vi "GUID.vi"() -> (3 "trimmed string":string caption="GUID")   [LabVIEW 2018]
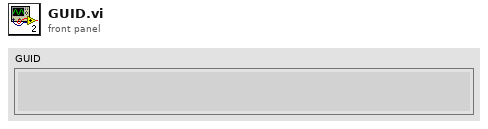
[diagram p1: front panel]
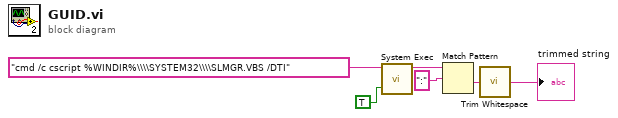
[diagram p0: block diagram]
diagram:
  n1 = call <vilib>:"System Exec.vi"("run minimized? (F)"=TRUE, "command line"="cmd /c cscript %WINDIR%\\\\SYSTEM32\\\\SLMGR.VBS /DTI") -> ("standard output"=w4:string)  [unwired: 6 in, 3 out]
  n2 = Match Pattern(string=w4, regular expression=":" ("正则表达式")) -> (after substring=w2:string)  [unwired: 1 in, 3 out]
  n3 = call <vilib>:"Trim Whitespace.vi"("string"=w2) -> ("trimmed string"=→"trimmed string":string)  [unwired: 1 in]
